vi "ex 2 - xor.vi"() -> ()   [LabVIEW 2016]
panel:
  out "Output":bool
  in  "Input 2":bool
  in  "Input 1":bool
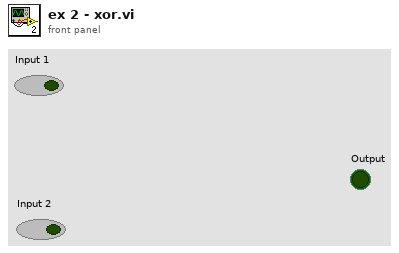
[diagram p1: front panel]
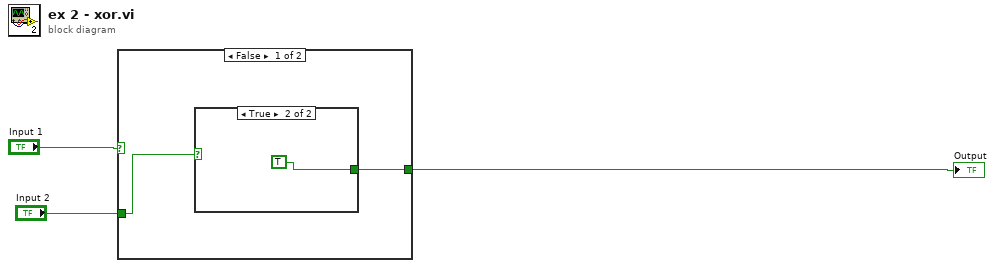
[diagram p0: block diagram]
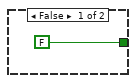
[diagram p2: hidden frame]
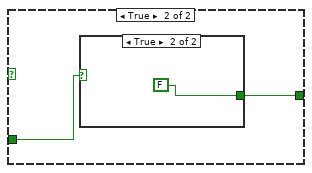
[diagram p3: hidden frame]
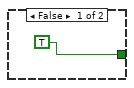
[diagram p4: hidden frame]
diagram:
  n1 = case shown="False" "Input 1" {
    tunnel: [w5 w9] -> w2
    tunnel: "Input 2" -> [w4 w8]
    frame False {
      n2 = case shown="True" w4 {
        tunnel: [FALSE TRUE] -> w5
        frame False {
        }
        frame True {
        }
      }
    }
    frame True {
      n3 = case shown="True" w8 {
        tunnel: [TRUE FALSE] -> w9
        frame False {
        }
        frame True {
        }
      }
    }
  }
  "Output" <- w2
